vi "PublishAllOpStates.vi"(7 "OpState tags":variant, 8 "error in (no error)":errorcluster, 9 "operating states transition time":variant, 10 "operating states":variant, 11 "status":variant) -> (0 "error out":errorcluster, 3 "tag value":T1[](array[typedef]))   [LabVIEW 2017, in "OpState.lvlib"]
uses:
  <vilib>/addons/InsightCM/Devices/Shared/Common/OpState/OpState.lvlib
  <vilib>/addons/InsightCM/MessageBus/Base/controls/TagValueString.ctl
  <vilib>/addons/InsightCM/MessageBus/Base/controls/TsTagValueString.ctl
  <vilib>/addons/InsightCM/Devices/Shared/Common/OpState/controls/TriggerOperatingState.ctl
  <vilib>/addons/InsightCM/MessageBus/Base/controls/KeyValuePair.ctl
  <vilib>/addons/InsightCM/Devices/Shared/Common/Trigger/controls/TriggerCondition.ctl
  <vilib>/addons/InsightCM/MessageBus/Base/controls/Condition.ctl
  <vilib>/addons/InsightCM/Devices/Shared/Common/Trigger/Trigger.lvlib
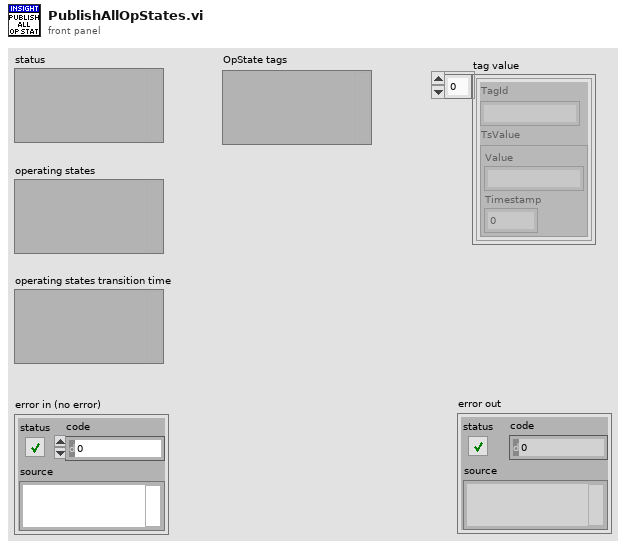
[diagram p1: front panel]
types:
  T1 = typedef "TagValueString.ctl" = cluster{"TagId":string, "TsValue":T2}
  T2 = typedef "TsTagValueString.ctl" = cluster{"Value":string, "Timestamp":i64}
  T3 = typedef "OpState.lvlib/TriggerOperatingState.ctl" = cluster{"Id":string, "Name":string, "Properties":T4[], "EnterExpression":string, "EnterConditions":T5[], "ExitExpression":string, "ExitConditions":T5[]}
  T4 = typedef "KeyValuePair.ctl" = cluster{"Key":string, "Value":string}
  T5 = typedef "Trigger.lvlib/TriggerCondition.ctl" = cluster{"Condition":T6, "LatchValue":string, "LatchTime":timestamp}
  T6 = typedef "Condition.ctl" = cluster{"Source":string, "Type":string, "Operator":string, "CompareTo":string, "DwellSeconds":dbl}
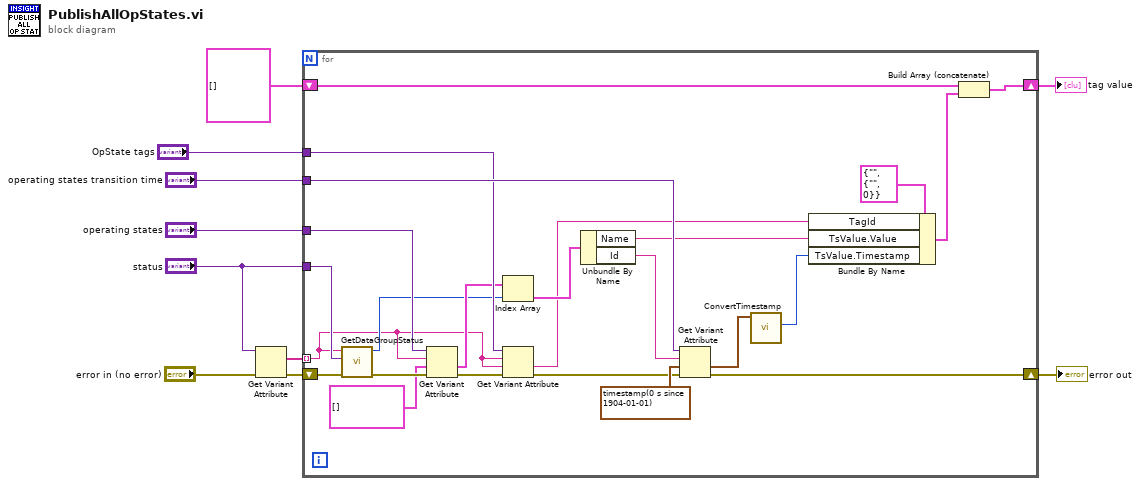
[diagram p0: block diagram]
diagram:
  n1 = Get Variant Attribute(Variant="status", error in="error in (no error)") -> (names=w9:string[], error out=w8:errorcluster)  [unwired: 2 in, 2 out]
  n2 = for {
    tunnel: w9 -> [w12] mode=indexing
    tunnel: "status" -> [w33]
    tunnel: "operating states" -> [w32]
    tunnel: "operating states transition time" -> [w29]
    shift-right: [w24] -> w1
    shift-left: T1[] [] ("tag value") -> [w26]
    shift-right: [w25] -> w4
    shift-left: w8 -> [w34]
    tunnel: "OpState tags" -> [w23]
    n3 = call <vilib>:"GetDataGroupStatus.vi"("error in"=w34, "status"=w33, "data group"=w12) -> ("error out"=w31:errorcluster, "CurrentOpState"=w21:i32)  [unwired: 7 in]
    n4 = Get Variant Attribute(Variant=w32, name=w12, default value (empty Variant)=T3[] [] ("OperatingStates"), error in=w31) -> (value=w22:T3[], error out=w28:errorcluster)  [unwired: 2 out]
    n5 = Index Array(array=w22, index=w21) -> (element=w14:T3)
    n6 = Get Variant Attribute(Variant=w23, name=w12, default value (empty Variant)=w12, error in=w28) -> (value=w11:string, error out=w17:errorcluster)  [unwired: 2 out]
    n7 = Unbundle By Name(w14) -> ("Name"=w13:string, "Id"=w16:string)
    n8 = Get Variant Attribute(Variant=w29, name=w16, default value (empty Variant)=timestamp(0 s since 1904-01-01) ("Time Stamp"), error in=w17) -> (value=w18:timestamp, error out=w25:errorcluster)  [unwired: 2 out]
    n9 = call <vilib>:"ConvertTimestamp.vi"("Time Stamp"=w18) -> ("Timestamp out"=w20:i64)  [unwired: 10 in]
    n10 = Bundle By Name(cluster=T1 {"TagId"="", "TsValue"={"Value"="", "Timestamp"=0}} ("TagValue"), "TagId"=w11, "TsValue.Value"=w13, "TsValue.Timestamp"=w20) -> (w27:T1)
    n11 = Build Array (concatenate)(w26, w27) -> (w24:T1[])
  }
  "error out" <- w4
  "tag value" <- w1
